vi "Load File.vi"(8 "error in (no error)":errorcluster, 10 "Item Configurations":refnum<class "Item Configuration.lvclass">[](array[class]), 11 "File Path":path) -> (0 "error out":errorcluster)   [LabVIEW 2013, in "File IO.lvlib"]
uses:
  File IO.lvlib
  Item Configuration/Item Configuration/Item Configuration.lvclass
  <vilib>/xml/Load XML File.vi
  <vilib>/xml/Close Reference(Node).vi
  <vilib>/xml/NI_XML.lvlib
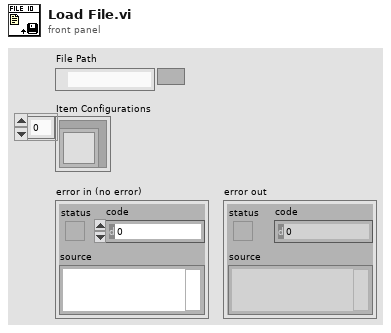
[diagram p1: front panel]
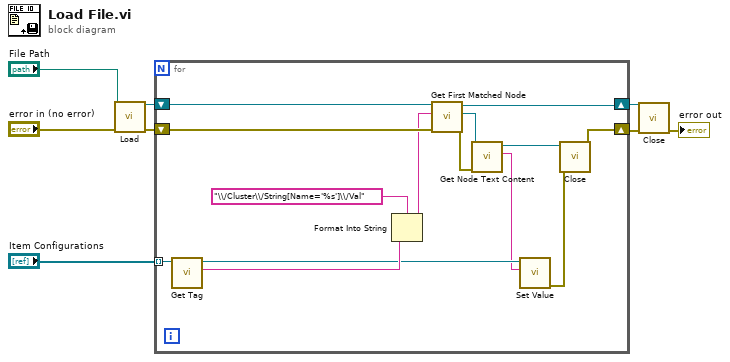
[diagram p0: block diagram]
diagram:
  n1 = call-poly <vilib>:"Load.vi"("path to XML document"="File Path", "error in (no error)"="error in (no error)") -> ("DOM document out"=w8:refnum<k20>, "error out"=w6:errorcluster)  [unwired: 11 in, 1 out]
  n2 = for {
    shift-right: [w22] -> w5
    shift-left: w8 -> [w21]
    shift-right: [w9] -> w4
    shift-left: w6 -> [w20]
    tunnel: "Item Configurations" -> [w16] mode=indexing
    n3 = call-dynamic "Get Tag.vi"("Item Configuration in"=w16) -> ("Project Info Tag"=w18:string, "Item Configuration out"=w13:refnum<class "Item Configuration.lvclass">)  [unwired: 8 in, 1 out]
    n4 = Format Into String(format string="\\/Cluster\\/String[Name='%s']\\/Val" ("XPath expression"), w18) -> (resulting string=w17:string)  [unwired: 2 in, 1 out]
    n5 = call <vilib>:"Get First Matched Node.vi"("error in (no error)"=w20, "XPath expression"=w17, "node in"=w21) -> ("error out"=w14:errorcluster, "node result"=w15:refnum<k20>, "node out"=w22:refnum<k20>)  [unwired: 6 in]
    n6 = call <vilib>:"Get Node Text Content.vi"("error in (no error)"=w14, "node in"=w15) -> ("node text"=w12:string, "node out"=w11:refnum<k20>)  [unwired: 7 in, 1 out]
    n7 = call-dynamic "Set Value.vi"("Project Info Value"=w12, "Item Configuration in"=w13) -> ("error out"=w10:errorcluster)  [unwired: 8 in, 1 out]
    n8 = call-poly <vilib>:"Close.vi"("error in (no error)"=w10, "node"=w11) -> ("error out"=w9:errorcluster)  [unwired: 7 in]
  }
  n9 = call-poly <vilib>:"Close.vi"("error in (no error)"=w4, "node"=w5) -> ("error out"=→"error out":errorcluster)  [unwired: 7 in]
